vi "add or remove from checkbox table.vi"(7 "Enable group mode":T1, 8 "error in (no error)":errorcluster, 9 "device list to add remove":string[](array[string]), 10 "child devices":string[](array[string]), 11 "MulticolumnListbox ref":refnum<vi>) -> (3 "ItemSyms":i32[](array[numeric]))   [LabVIEW 2020]
uses:
  General-Controler/enable group typ def.ctl
  <userlib>/_OpenG.lib/array/array.llb/Conditional Auto-Indexing Tunnel (String)__ogtk.vi
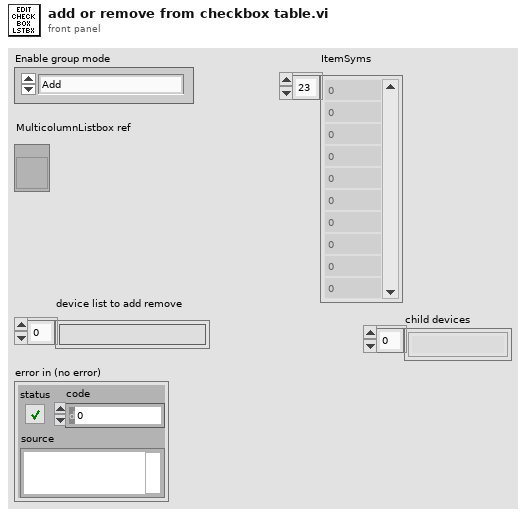
[diagram p1: front panel]
types:
  T1 = typedef "enable group typ def.ctl" = enum16{"Add", "Remove", "Add All", "Remove All"}
  T2 = typedef "mysql_authentication.ctl" = cluster{"User":string, "Password":string, "Database":string}
  T3 = cluster{"Port":u16, "IP Address":string, "Authentication":T2}
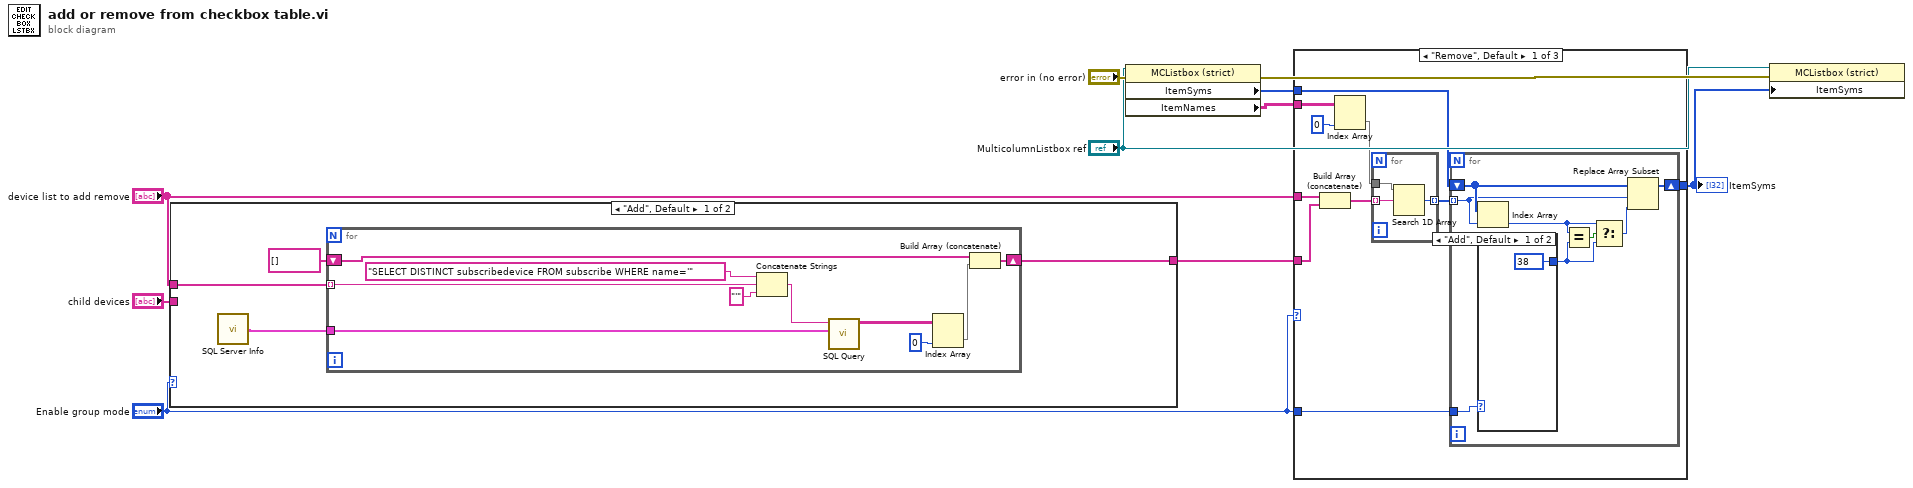
[diagram p0: block diagram]
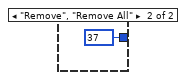
[diagram p2: hidden frame]
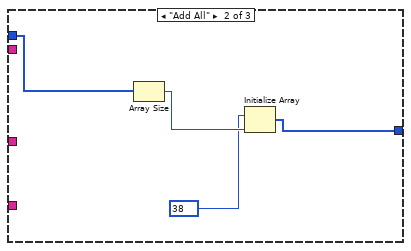
[diagram p3: hidden frame]
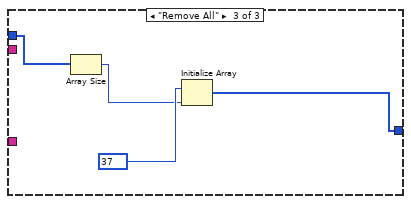
[diagram p4: hidden frame]
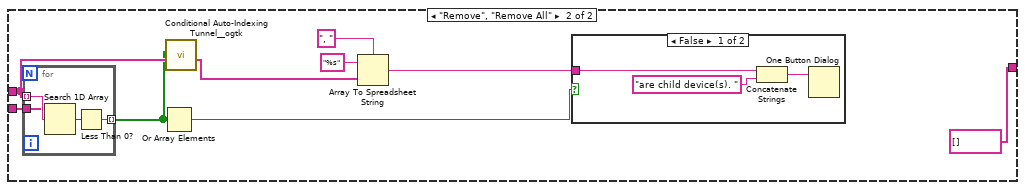
[diagram p5: hidden frame]
diagram:
  n1 = case shown="\"Add\", Default" "Enable group mode" {
    tunnel: "device list to add remove" -> [w14 w33]
    tunnel: [w12 string[] [] ("device list to add remove")] -> w9
    tunnel: "child devices" -> [_ w25]
    frame "Add", Default {
      n2 = call "SQL Server Info.vi"() -> ("SQL Server Info"=w11:T3)
      n3 = for {
        tunnel: w14 -> [w19] mode=indexing
        shift-right: [w16] -> w12
        shift-left: string[] [] ("device list to add remove") -> [w18]
        tunnel: w11 -> [w15]
        n4 = Concatenate Strings("SELECT DISTINCT subscribedevice FROM subscribe WHERE name='" ("Query"), w19, "'" ("string")) -> (w22:string)
        n5 = call "SQL Query.vi"("SQL Server Info"=w15, "Query"=w22) -> ("data"=w23:string[][])  [unwired: 8 in, 1 out]
        n6 = Index Array(array=w23, index (col)=0 ("disabled index (col)")) -> (element=w17:string[])  [unwired: 1 in]
        n7 = Build Array (concatenate)(w18, w17) -> (w16:string[])
      }
    }
    frame "Remove", "Remove All" {
      n8 = for {
        tunnel: [w35] -> w28 mode=indexing
        tunnel: w33 -> [w36] mode=indexing
        tunnel: w25 -> [w34]
        n9 = Search 1D Array(1D array=w34, element=w36) -> (index of element=w37:i32)  [unwired: 1 in]
        n10 = Less Than 0?(x=w37) -> (x < 0?=w35:bool)
      }
      n11 = Or Array Elements(Boolean array=w28) -> (logical OR=w27:bool)
      n12 = call-poly <userlib>:"Conditional Auto-Indexing Tunnel__ogtk.vi"("Array in"=w33, "Elements to keep"=w28) -> ("Filtered Array out"=w32:string[])  [unwired: 5 in]
      n13 = Array To Spreadsheet String(delimiter (Tab)=", ", array=w32, 3:"%s" ("format string")) -> (spreadsheet string=w29:string)
      n14 = case shown="False" w27 {
        tunnel: w29 -> [w39 _]
        frame False {
          n15 = Concatenate Strings(w39, "are child device(s). " ("message")) -> (w38:string)
          n16 = One Button Dialog(message=w38) -> ()  [unwired: 1 in, 1 out]
        }
        frame True {
        }
      }
    }
  }
  n17 = property on="Property Node" class="MCListbox (strict)"(reference="MulticolumnListbox ref", error in="error in (no error)") -> (error out=w4:errorcluster, "ItemSyms"=w6:i32[], "ItemNames"=w5:string[][])  [unwired: 1 out]
  n18 = case shown="\"Remove\", Default" "Enable group mode" {
    tunnel: "device list to add remove" -> [w50 _ _]
    tunnel: w9 -> [w48 _ _]
    tunnel: "Enable group mode" -> [w47 _ _]
    tunnel: [w46 w64 w68] -> w8
    tunnel: w6 -> [w45 w66 w70]
    tunnel: w5 -> [w44 _ _]
    frame "Remove", Default {
      n19 = Build Array (concatenate)(w50, w48) -> (w49:string[])
      n20 = Index Array(array=w44, index (col)=0 ("disabled index (col)")) -> (element=w41:string[])  [unwired: 1 in]
      n21 = for {
        tunnel: w49 -> [w62] mode=indexing
        tunnel: w41 -> [w63]
        tunnel: [w61] -> w43 mode=indexing
        n22 = Search 1D Array(1D array=w63, element=w62) -> (index of element=w61:i32)  [unwired: 1 in]
      }
      n23 = for {
        shift-right: [w53] -> w46
        shift-left: w45 -> [w56]
        tunnel: w43 -> [w55] mode=indexing
        tunnel: w47 -> [w51]
        n24 = Index Array(array=w56, index=w55) -> (element=w52:i32)
        n25 = case shown="\"Add\", Default" w51 {
          tunnel: [38 37] -> w57
          frame "Add", Default {
          }
          frame "Remove", "Remove All" {
          }
        }
        n26 = Equal?(x=w52, y=w57) -> (x = y?=w58:bool)
        n27 = Select(t=w52, s=w58, f=w57) -> (s? t:f=w54:i32)
        n28 = Replace Array Subset(array=w56, new element=w54, index=w55) -> (w53:i32[])
      }
    }
    frame "Add All" {
      n29 = Array Size(array=w66) -> (size(s)=w67:i32)
      n30 = Initialize Array(38, w67) -> (w64:i32[])
    }
    frame "Remove All" {
      n31 = Array Size(array=w70) -> (size(s)=w69:i32)
      n32 = Initialize Array(37, w69) -> (w68:i32[])
    }
  }
  "ItemSyms" <- w8
  n33 = property on="Property Node" class="MCListbox (strict)"(reference="MulticolumnListbox ref", error in=w4, "ItemSyms"=w8) -> ()  [unwired: 2 out]
